vi "version.vi"() -> ()   [LabVIEW 2014]
panel:
  in  "VER":string
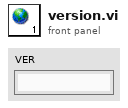
[diagram p1: front panel]
diagram:
